vi "guess.validate.vi"(11 "Worder in":refnum<class "Worder.lvclass">) -> (3 "valid?":bool)   [LabVIEW 2020, in "Worder.lvclass"]
uses:
  Worder.lvclass
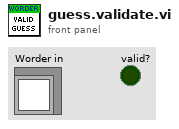
[diagram p1: front panel]
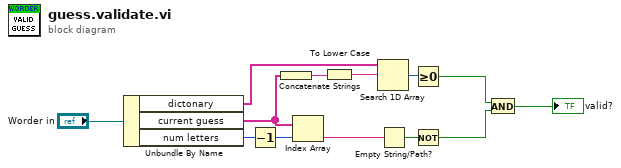
[diagram p0: block diagram]
diagram:
  n1 = Unbundle By Name("Worder in") -> ("dictonary"=w7:string[], "current guess"=w8:string[], "num letters"=w12:i32)
  n2 = Decrement(x=w12) -> (x-1=w11:i32)
  n3 = Concatenate Strings(w8) -> (w4:string)
  n4 = Index Array(array=w8, index=w11) -> (element=w9:string)
  n5 = To Lower Case(string=w4) -> (all lower case string=w3:string)
  n6 = Search 1D Array(1D array=w7, element=w3) -> (index of element=w6:i32)  [unwired: 1 in]
  n7 = Empty String/Path?(string/path=w9) -> (empty?=w10:bool)
  n8 = Greater Or Equal To 0?(x=w6) -> (x >= 0?=w5:bool)
  n9 = Not(x=w10) -> (.not. x?=w2:bool)
  n10 = And(x=w5, y=w2) -> (x .and. y?=→"valid?":bool)
